vi "ResetHints.vi"(8 "No Error":errorcluster) -> (0 "error out":errorcluster)   [LabVIEW 2026, in "SDL3.lvlib" / "Hints.lvlib"]
doc: "<B>Summary</B>\nReset all hints to the default values.\n\n<B>Remarks</B>\nThis will reset all hints to the value of the associated environment variable, or NULL if the environment isn't set. Callbacks will be called normally with this change."
uses:
  Hints.lvlib
  Lib/SDL3.dll
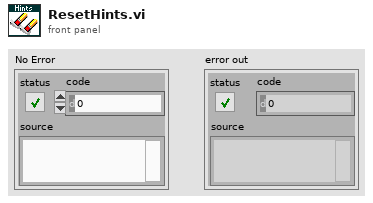
[diagram p1: front panel]
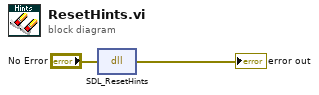
[diagram p0: block diagram]
diagram:
  n1 = dll-call lib="C:/Users/saukko/Dev/LV-SDL3/Sources/SDL3/Lib/SDL3.*" fn="SDL_ResetHints"(error in="No Error") -> (error out=→"error out":errorcluster)  [unwired: 3 in, 1 out]
